vi "KEYS.vi"(8 "error in (no error)":errorcluster, 10 "pattern":string="*", 11 "Redis Client in":refnum<class "Redis Client.lvclass">) -> (0 "error out":errorcluster, 2 "keys":set{string}(c389), 3 "Redis Client out":refnum<class "Redis Client.lvclass">)   [LabVIEW 2023, in "Redis Client for LabVIEW.lvlib" / "Redis Client.lvclass"]
uses:
  Redis Client.lvclass
  lib/RESP3-for-LabVIEW/RESP3/subVIs/RESP3 Make String Base.vi
  lib/RESP3-for-LabVIEW/RESP3/types/RESP3 data type attribute.vi
  lib/RESP3-for-LabVIEW/RESP3/high-level/RESP3 Get Array.vi
  lib/RESP3-for-LabVIEW/RESP3/high-level/RESP3 Get String.vi
  Redis Client.lvclass/Redis Client.ctl
  lib/RESP3-for-LabVIEW/RESP3/RESP3.lvlib
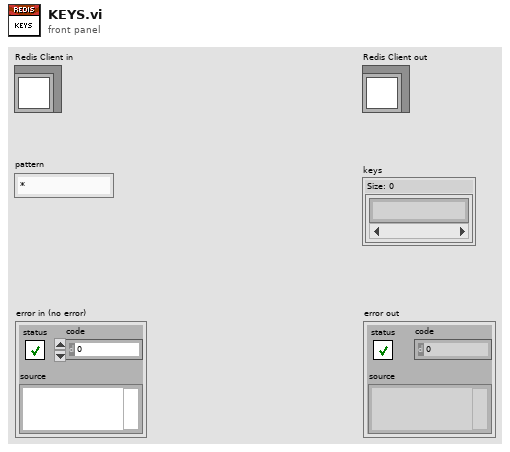
[diagram p1: front panel]
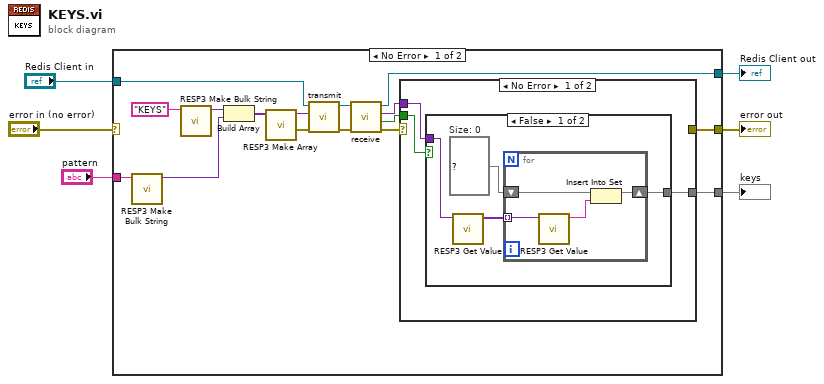
[diagram p0: block diagram]
diagram:
  n1 = case shown="No Error" "error in (no error)" {
    selector: "error in (no error)" -> [_ w36]
    tunnel: [w20 w36] -> w5
    tunnel: "Redis Client in" -> [w22 w35]
    tunnel: [w7 w35] -> w3
    tunnel: "pattern" -> [w17 _]
    tunnel: [w19 _] -> w1
    frame No Error {
      n2 = call "RESP3 Make Bulk String.vi"("String"=w17) -> ("RESP3 Value out"=w16:variant)  [unwired: 9 in, 1 out]
      n3 = call "RESP3 Make Bulk String.vi"("String"="KEYS" ("string in")) -> ("RESP3 Value out"=w15:variant)  [unwired: 9 in, 1 out]
      n4 = Build Array(w15, w16) -> (w21:variant[])
      n5 = call "RESP3 Make Array.vi"("RESP3 Values in"=w21) -> ("error out"=w13:errorcluster, "RESP3 Value out"=w14:variant)  [unwired: 9 in]
      n6 = call-dynamic "transmit.vi"("error in (no error)"=w13, "RESP3 Value"=w14, "Redis Client in"=w22) -> ("error out"=w11:errorcluster, "Redis Client out"=w12:refnum<class "Redis Client.lvclass">)  [unwired: 7 in]
      n7 = call-dynamic "receive.vi"("error in (no error)"=w11, "Redis Client in"=w12) -> ("error out"=w10:errorcluster, "timed out?"=w8:bool, "RESP3 Value"=w9:variant, "Redis Client out"=w7:refnum<class "Redis Client.lvclass">)  [unwired: 6 in]
      n8 = case shown="No Error" w10 {
        selector: w10 -> [_ w34]
        tunnel: [_ w34] -> w20
        tunnel: [w25 _] -> w19
        tunnel: w9 -> [w23 _]
        tunnel: w8 -> [w24 _]
        frame No Error {
          n9 = case shown="False" w24 {
            tunnel: [w29 _] -> w25
            tunnel: w23 -> [w28 _]
            frame False {
              w26 = set{string} {}  # Size: 0
              n10 = call-poly "RESP3 Get Value.vi"("RESP3 Value in"=w28) -> ("RESP3 Values out"=w27:variant[])  [unwired: 7 in, 3 out]
              n11 = for {
                shift-right: [w33] -> w29
                shift-left: w26 -> [w32]
                tunnel: w27 -> [w31] mode=indexing
                n12 = call-poly "RESP3 Get Value.vi"("RESP3 Value in"=w31) -> ("String out"=w30:string)  [unwired: 7 in, 3 out]
                n13 = Insert Into Set(10:w30, 11:w32) -> (3:w33:set{string})  [unwired: 1 out]
              }
            }
            frame True {
            }
          }
        }
        frame Error {
        }
      }
    }
    frame Error {
    }
  }
  "error out" <- w5
  "Redis Client out" <- w3
  "keys" <- w1
